vi "Prova lettura perdite di carico.vi"() -> ()   [LabVIEW 2019]
panel:
  out "error out 2":errorcluster
  in  "Enum":T1(ring)
  in  "Excel._Worksheet 2":refnum<k7>
  out "Perdite carico ASP":dbl
  out "Perdite carico MAND":dbl
  in  "WindowState 2":i32(ring)=-4140 items=["xlMaximized"=-4137, "xlMinimized"=-4140, "xlNormal"=-4143]
  out "error out":errorcluster
  in  "path":path
  in  "stop":bool
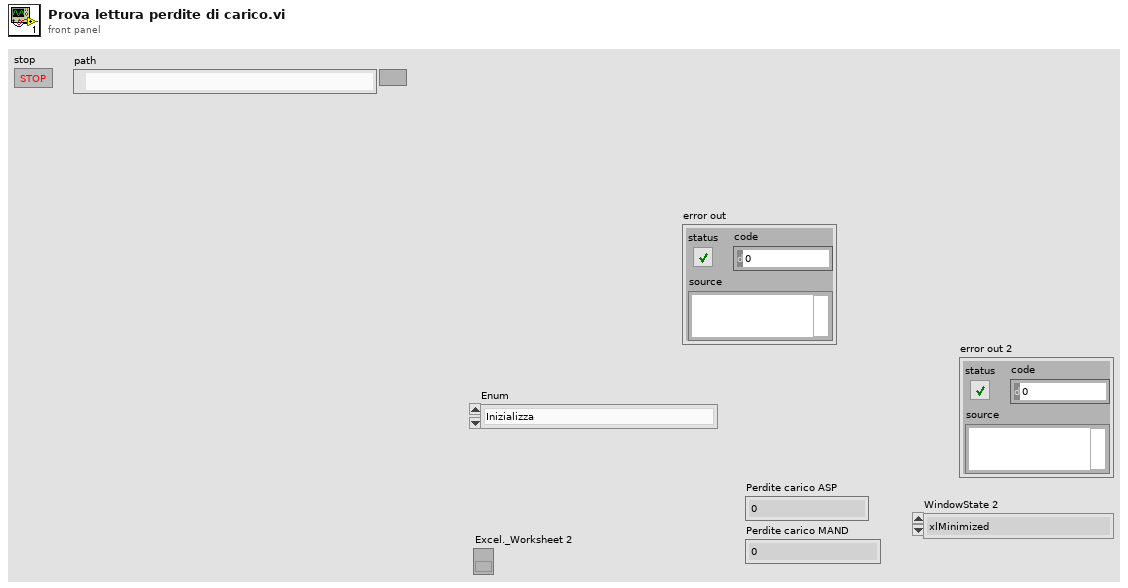
[diagram p1: front panel]
types:
  T1 = enum16{"Inizializza", "Imposta selezioni pompa", "Leggi perdite", "Close"}
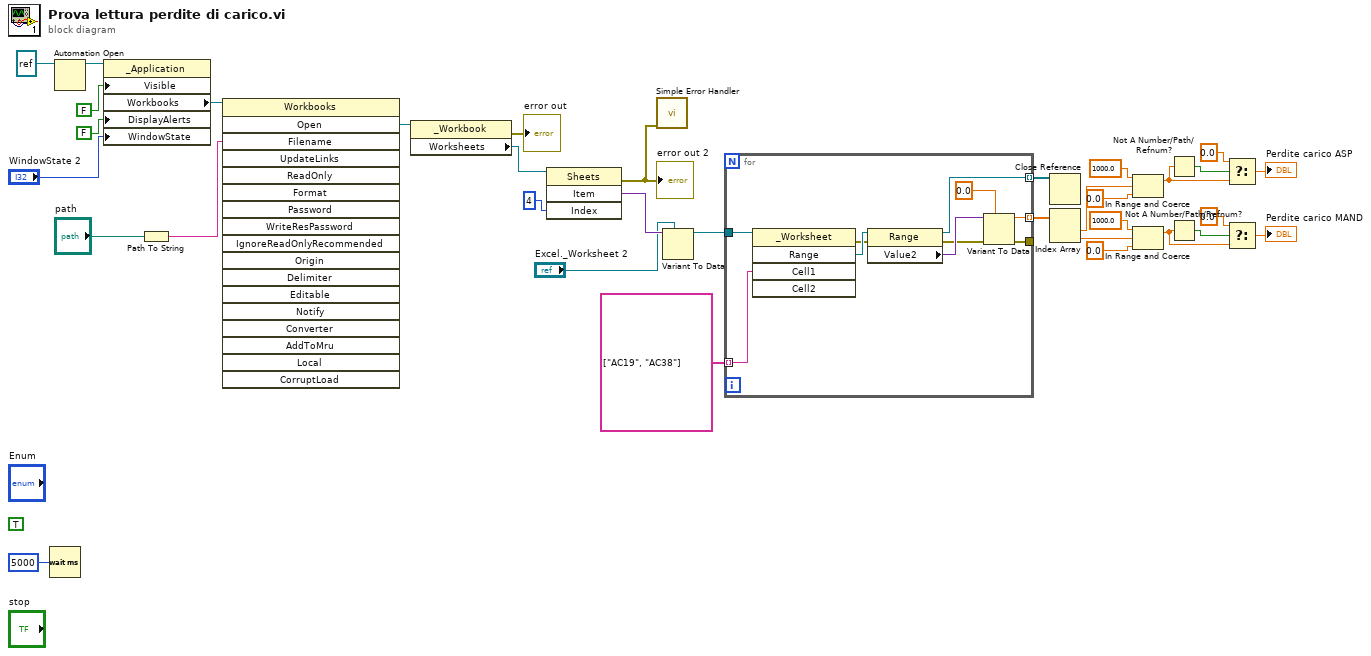
[diagram p0: block diagram]
diagram:
  (unwired) TRUE
  n1 = Wait (ms)(milliseconds to wait=u32 5000) -> ()  [unwired: 1 out]
  n2 = Automation Open(Automation Refnum=refnum<k7> refnum ("Excel._Application")) -> (Automation Refnum=w11:refnum<k7>)  [unwired: 3 in, 1 out]
  n3 = property class="_Application"(reference=w11, "Visible"=FALSE, "DisplayAlerts"=FALSE, "WindowState"="WindowState 2") -> ("Workbooks"=w9:refnum<k7>)  [unwired: 1 in, 2 out]
  n4 = Path To String(path="path") -> (string=w10:string)
  n5 = invoke class="Workbooks" method="Open"(reference=w9, "Filename"=w10) -> ("Open"=w12:refnum<k7>)  [unwired: 16 in, 17 out]
  n6 = property class="_Workbook"(reference=w12) -> (error out=→"error out":errorcluster, "Worksheets"=w2:refnum<k7>)  [unwired: 1 in, 1 out]
  n7 = invoke class="Sheets" method="Item"(reference=w2, "Index"=4) -> (error out=w34:errorcluster, "Item"=w16:variant)  [unwired: 2 in, 2 out]
  "error out 2" <- w34
  n8 = call <vilib>:"Simple Error Handler.vi"("error in (no error)"=w34) -> ()  [unwired: 4 in, 5 out]
  n9 = Variant To Data(type="Excel._Worksheet 2", Variant=w16) -> (data=w14:refnum<k7>)  [unwired: 1 in, 1 out]
  n10 = for {
    tunnel: w14 -> [w44]
    tunnel: [w39] -> w19 mode=indexing
    tunnel: string[] ["AC19", "AC38"] -> [w38] mode=indexing
    tunnel: [w36] -> _
    tunnel: [w35] -> w18 mode=indexing
    n11 = invoke class="_Worksheet" method="Range"(reference=w44, "Cell1"=w38) -> (error out=w42:errorcluster, "Range"=w43:refnum<k7>)  [unwired: 3 in, 3 out]
    n12 = property class="Range"(reference=w43, error in=w42) -> (reference out=w35:refnum<k7>, error out=w40:errorcluster, "Value2"=w41:variant)
    n13 = Variant To Data(error in=w40, type=0.0, Variant=w41) -> (data=w39:dbl, error out=w36:errorcluster)
  }
  n14 = Close Reference(reference=w18) -> ()  [unwired: 1 in, 1 out]
  n15 = Index Array(array=w19) -> (element #1=w20:dbl, element #2=w25:dbl)  [unwired: 2 in]
  n16 = In Range and Coerce(upper limit=1000.0, x=w20, lower limit=0.0) -> (coerced(x)=w28:dbl)  [unwired: 1 out]
  n17 = In Range and Coerce(upper limit=1000.0, x=w25, lower limit=0.0) -> (coerced(x)=w32:dbl)  [unwired: 1 out]
  n18 = Not A Number/Path/Refnum?(number/path/refnum=w28) -> (NaN/Path/Refnum?=w26:bool)
  n19 = Not A Number/Path/Refnum?(number/path/refnum=w32) -> (NaN/Path/Refnum?=w31:bool)
  n20 = Select(t=0.0, s=w26, f=w28) -> (s? t:f=→"Perdite carico ASP":dbl)
  n21 = Select(t=0.0, s=w31, f=w32) -> (s? t:f=→"Perdite carico MAND":dbl)
